vi "subtract.vi"(10 "x":dbl, 11 "y":dbl) -> (2 "x-y":dbl)   [LabVIEW 2018]
panel:
  in  "Slide":dbl(slide) scale=0.0..10.0
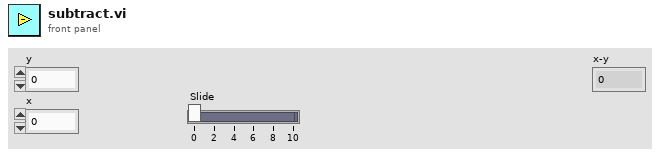
[diagram p1: front panel]
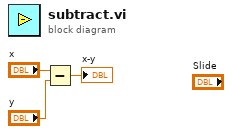
[diagram p0: block diagram]
diagram:
  n1 = Subtract(x="x", y="y") -> (x-y=→"x-y":dbl)
